vi "Read Module Vacuum.vi"(8 "error in":errorcluster, 9 "Slot Number":i32, 10 "Chuck Number":i32, 11 "Gantry in":refnum<class "Gantry Class.lvclass">) -> (0 "error out":errorcluster, 2 "On/Off":bool, 3 "Gantry out":refnum<class "Gantry Class.lvclass">)   [LabVIEW 2011, in "Gantry Class.lvclass"]
uses:
  Gantry Class.lvclass
  WorkTable Class/WorkTable Class.lvclass
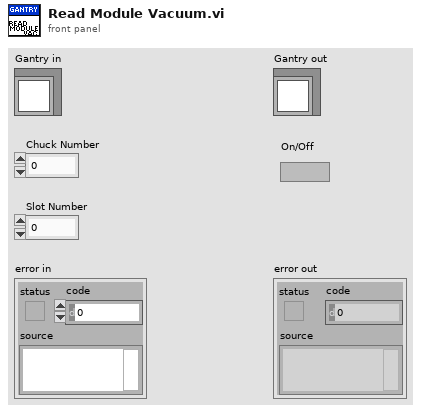
[diagram p1: front panel]
types:
  T1 = typedef "Worktable_Module Slot.ctl" = cluster{"Slot State":enum16{"Empty", "Bare HDI", "Unglued", "Stamped", "PartOnTop", "Weighted", "Unpotted", "Potted"}, "BBM Type":enum16{"None", "BBM", "GlassSlide"}, "HDI Type":enum16{"None", "HDI", "Polyimide"}, "Vacuum Channel":u8, "Location/Orientation BBM":T2, "Location/Orientation HDI":T2, "S/N":string}
  T2 = typedef "Position_Orientation.ctl" = cluster{"Center":refnum<class "Vec3d Class.lvclass">, "Orientation":refnum<class "Orient3d Class.lvclass">}
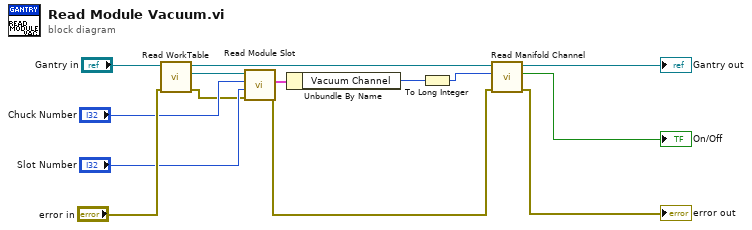
[diagram p0: block diagram]
diagram:
  n1 = call-dynamic "Read WorkTable.vi"("error in"="error in", "Gantry Class in"="Gantry in") -> ("error out"=w3:errorcluster, "WorkTable Class.lvclass"=w7:refnum<class "WorkTable Class.lvclass">, "Gantry Class out"=w4:refnum<class "Gantry Class.lvclass">)  [unwired: 7 in]
  n2 = call-dynamic "Read Module Slot.vi"("error in"=w3, "slot"="Slot Number", "chuck"="Chuck Number", "WorkTable in"=w7) -> ("error out"=w5:errorcluster, "Module Slot"=w6:T1)  [unwired: 5 in, 1 out]
  n3 = Unbundle By Name(w6) -> ("Vacuum Channel"=w2:u8)
  n4 = To Long Integer(number=w2) -> (32bit integer=w1:i32)
  n5 = call-dynamic "Read Manifold Channel.vi"("error in"=w5, "Manifold Channel"=w1, "Gantry in"=w4) -> ("error out"=→"error out":errorcluster, "On/Off"=→"On/Off":bool, "Gantry out"=→"Gantry out":refnum<class "Gantry Class.lvclass">)  [unwired: 6 in]
